vi "Calculate INL.vi"(10 "DNL":dbl[](array[numeric])) -> (1 "Max INL":i32, 2 "INL":dbl, 3 "INL waveform":dbl[](array[numeric]))   [LabVIEW 2021, in "Linearity_DAC.lvlib"]
uses:
  Linearity_DAC.lvlib
  <vilib>/Analysis/NI_AALPro.lvlib
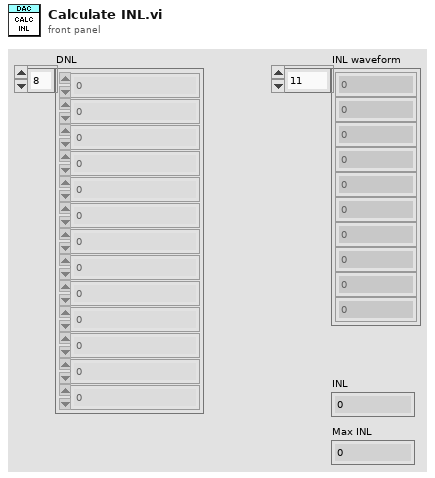
[diagram p1: front panel]
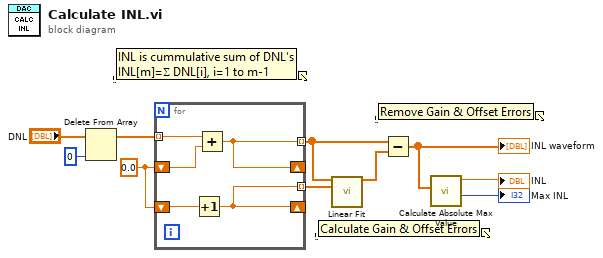
[diagram p0: block diagram]
diagram:
  w10 = 0.0
  n1 = Delete From Array(array="DNL", index=0) -> (array with subset deleted=w2:dbl[])  [unwired: 1 in, 1 out]
  n2 = for {
    tunnel: w2 -> [w15] mode=indexing
    shift-right: [w13] -> _
    shift-left: w10 -> [w14]
    tunnel: [w13] -> w5 mode=indexing
    shift-right: [w11] -> _
    shift-left: w10 -> [w12]
    tunnel: [w11] -> w9 mode=indexing
    n3 = Increment(x=w12) -> (x+1=w11:dbl)
    n4 = Add(x=w15, y=w14) -> (x+y=w13:dbl)
  }
  n5 = call <vilib>:"Linear Fit.vi"("Y"=w5, "X"=w9) -> ("Best Linear Fit"=w4:dbl[])  [unwired: 9 in, 4 out]
  n6 = Subtract(x=w5, y=w4) -> (x-y=w8:dbl[])
  "INL waveform" <- w8
  n7 = call "Calculate Absolute Max Value.vi"("Data"=w8) -> ("Abs max index"=→"Max INL":i32, "Abs max value"=→"INL":dbl)  [unwired: 9 in]
